vi "Trajectory_Creation_Pathfinder_Create.vi"() -> (0 "Path calculation error":errorcluster, 1 "Relative Trajectory":T1 {"States"."POSE"."ROTATION"."SIN" format="%13.4f"; "States"."POSE"."ROTATION"."COS" format="%13.4f"; "States"."POSE"."ROTATION"."VALUE" format="%13.4f"; "States"."POSE"."TRANSLATION"."Y" format="%14.3f"; "States"."POSE"."TRANSLATION"."X" format="%14.3f"; "TotalTImeSecs" format="%20.3f"}, 2 "Trajectory Items":i32, 3 "TotalTImeSecs":dbl)   [LabVIEW 2019]
uses:
  <vilib>/Rock Robotics/WPI/ThirdParty/JBRUN/PathFinder/VIs/Waypoint.ctl
  <vilib>/Rock Robotics/WPI/ThirdParty/JAS_Junk/TrajLib/TypeDef/TRAJECTORY.ctl
  <vilib>/Rock Robotics/WPI/ThirdParty/JAS_Junk/TrajLib/TypeDef/TRAJ_STATE.ctl
  <vilib>/Rock Robotics/WPI/ThirdParty/JAS_Junk/TrajLib/TypeDef/POSE2D.ctl
  <vilib>/Rock Robotics/WPI/ThirdParty/JAS_Junk/TrajLib/TypeDef/TRANSLATION2D.ctl
  <vilib>/Rock Robotics/WPI/ThirdParty/JAS_Junk/TrajLib/TypeDef/ROTATION2D.ctl
  <vilib>/Rock Robotics/WPI/ThirdParty/JAS_Junk/TrajLib/Trajectory_Library.lvlib
  <vilib>/Rock Robotics/WPI/ThirdParty/JBRUN/PathFinder/Pathfinder.lvlib
panel:
  out "Trajectory":cluster{dbl[], dbl[]}[](graph)
  in  "Waypoints":T6[](array[typedef])=[{"x"=15.0, "y"=105.0, "angle"=-45.0}, {"x"=105.0, "y"=65.0, "angle"=0.0}, {"x"=210.0, "y"=106.0, "angle"=45.0}]
  in  "wheelbase_width  IN":dbl=20.866
  in  "sample_count":i32=10000
  in  "Path Results\ndT":dbl=0.02 format="%7.3f"
  in  "max_jerk  IN/Sec^3":dbl=50.0
  in  "max_acceleration IN/Sec^2":dbl=20.0
  in  "max_velocity  IN/SEC":dbl=40.0
  # "TRAJECTORY CONFIGURATION"
  # "TRAJECTORY DEFINITION"
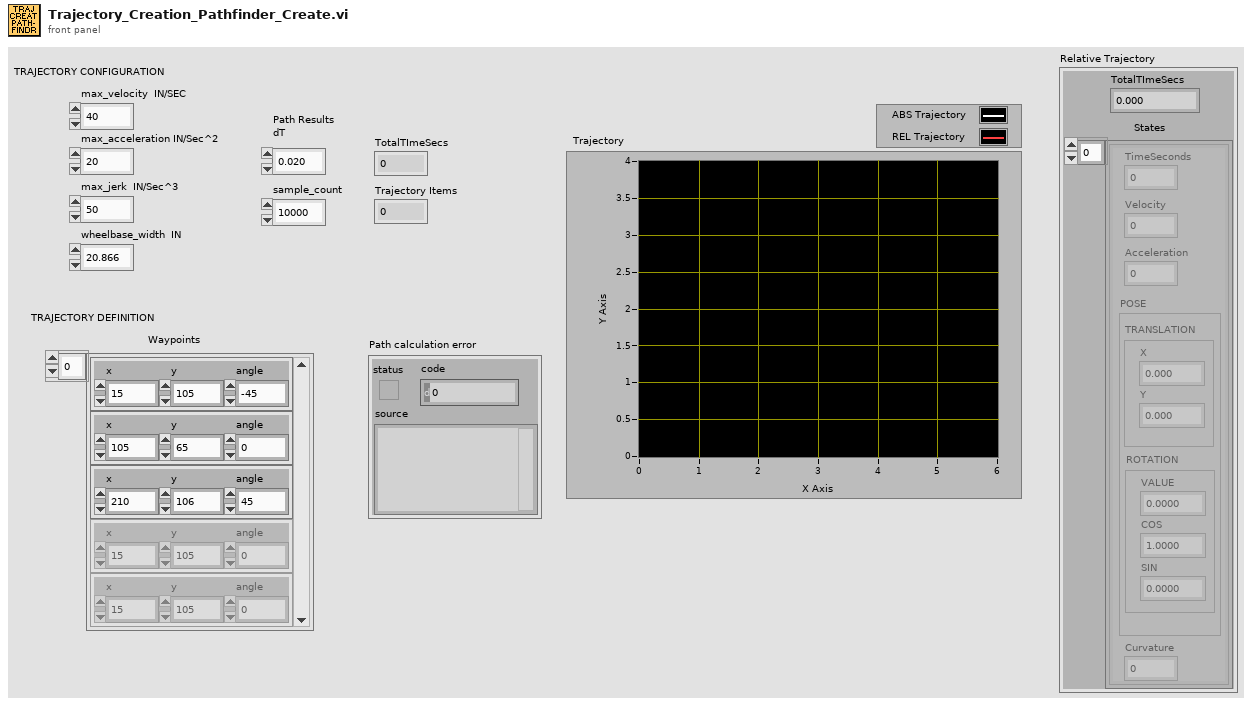
[diagram p1: front panel]
types:
  T1 = typedef "Trajectory_Library.lvlib/TRAJECTORY.ctl" = cluster{"TotalTImeSecs":dbl, "States":T2[]}
  T2 = typedef "Trajectory_Library.lvlib/TRAJ_STATE.ctl" = cluster{"TimeSeconds":dbl, "Velocity":dbl, "Acceleration":dbl, "POSE":T3, "Curvature":dbl}
  T3 = typedef "Trajectory_Library.lvlib/POSE2D.ctl" = cluster{"TRANSLATION":T4, "ROTATION":T5}
  T4 = typedef "Trajectory_Library.lvlib/TRANSLATION2D.ctl" = cluster{"X":dbl, "Y":dbl}
  T5 = typedef "Trajectory_Library.lvlib/ROTATION2D.ctl" = cluster{"VALUE":dbl, "COS":dbl, "SIN":dbl}
  T6 = typedef "Pathfinder.lvlib/Waypoint.ctl" = cluster{"x":dbl, "y":dbl, "angle":dbl}
  T7 = typedef "Pathfinder.lvlib/Segment.ctl" = cluster{"dt":dbl, "x":dbl, "y":dbl, "position":dbl, "velocity":dbl, "acceleration":dbl, "jerk":dbl, "heading":dbl}
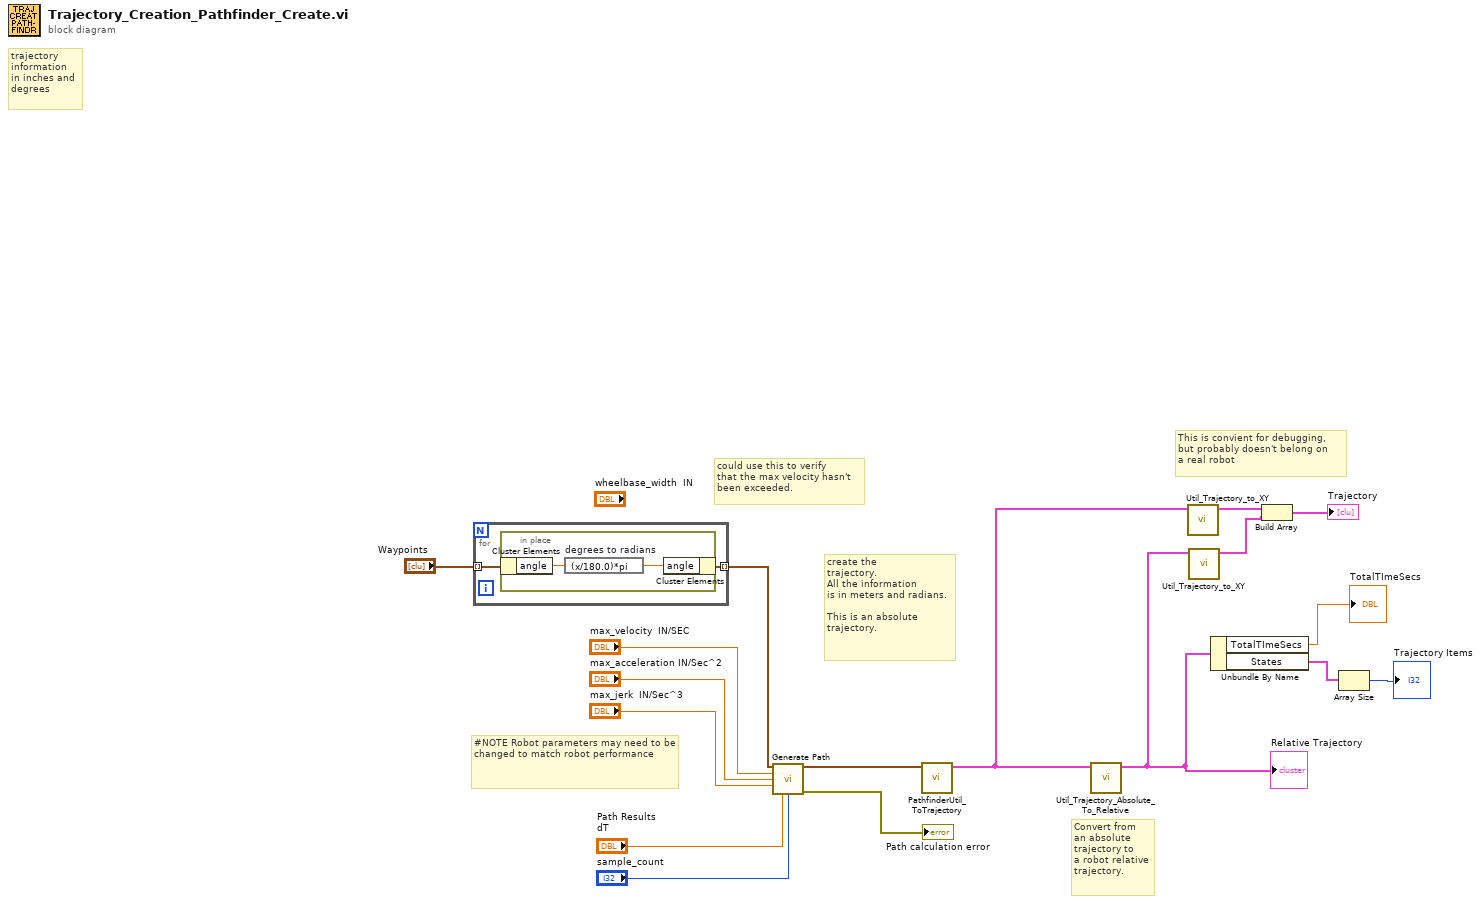
[diagram p0: block diagram]
diagram:
  # "This is convient for debugging,\nbut probably doesn't belong on\na real robot"
  # "#NOTE Robot parameters may need to be changed to match robot performance"
  # "could use this to verify\nthat the max velocity hasn't\nbeen exceeded."
  # "Convert from\nan absolute\ntrajectory to\na robot relative\ntrajectory."
  # "create the\ntrajectory.\nAll the information\nis in meters and radians.\n\nThis is an absolute \ntrajectory."
  # "trajectory\ninformation\nin inches and\ndegrees"
  n1 = for {
    tunnel: "Waypoints" -> [w19] mode=indexing
    tunnel: [w18] -> w13 mode=indexing
    n2 = in-place {
      n3 = in-place-cluster #1(w19) -> ("angle"=w21:dbl)
      n4 = expression code="(x/180.0)*pi" "degrees to radians"(w21) -> (w20:dbl)
      n5 = in-place-cluster #1("angle"=w20) -> (w18:T6)
    }
  }
  n6 = call <vilib>:"Generate Path.vi"("path"=w13, "max_velocity"="max_velocity  IN/SEC", "max_acceleration"="max_acceleration IN/Sec^2", "max_jerk"="max_jerk  IN/Sec^3", "dt (.001)"="Path Results\ndT", "sample_count (100000)"="sample_count") -> ("Segments"=w7:T7[], "error out"=→"Path calculation error":errorcluster)  [unwired: 8 in]
  n7 = call <vilib>:"PathfinderUtil_ToTrajectory.vi"("Pathfinder Path"=w7) -> ("TRAJECTORY"=w1:T1)  [unwired: 10 in]
  n8 = call <vilib>:"Util_Trajectory_Absolute_To_Relative.vi"("absTRAJECTORY"=w1) -> ("outputRelativeTRAJECTORY"=w2:T1)  [unwired: 10 in]
  "Relative Trajectory" <- w2
  n9 = call <vilib>:"Util_Trajectory_to_XY.vi"("TRAJECTORY"=w1) -> ("outArrayXY"=w5:cluster{dbl[], dbl[]})  [unwired: 10 in]
  n10 = call <vilib>:"Util_Trajectory_to_XY.vi"("TRAJECTORY"=w2) -> ("outArrayXY"=w4:cluster{dbl[], dbl[]})  [unwired: 10 in]
  n11 = Unbundle By Name(w2) -> ("TotalTImeSecs"=→"TotalTImeSecs":dbl, "States"=w16:T2[])
  n12 = Build Array(w5, w4) -> (→"Trajectory":cluster{dbl[], dbl[]}[])
  n13 = Array Size(array=w16) -> (size(s)=→"Trajectory Items":i32)
